vi "RPM_to_Motor_Input_v1.vi"(1 "Right Motor?":bool, 2 "RPM":dbl=1000.0) -> (0 "Motor Input":dbl)   [LabVIEW 2012]
uses:
  <vilib>/gmath/NI_Gmath.lvlib
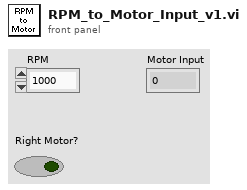
[diagram p1: front panel]
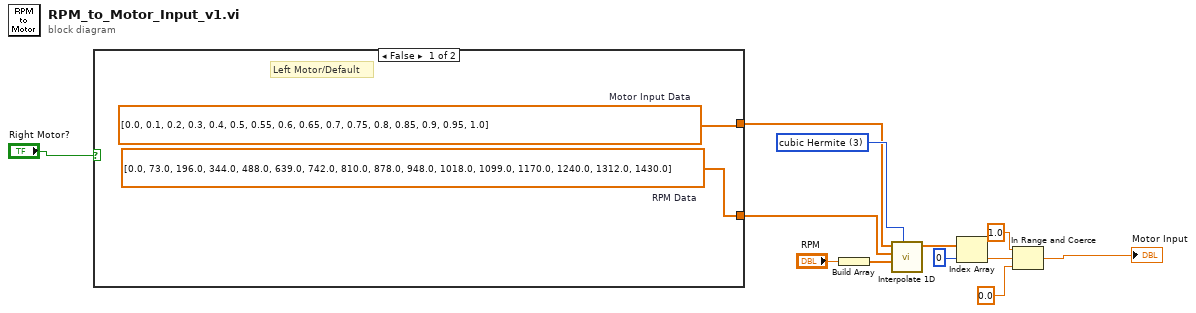
[diagram p0: block diagram]
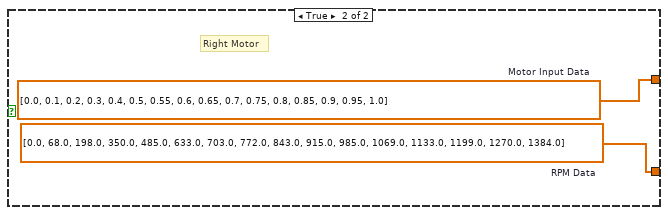
[diagram p2: hidden frame]
diagram:
  w8 = 3 items=["nearest", "linear", "spline", "cubic Hermite", "Lagrange"] ("method")
  n1 = case shown="False" "Right Motor?" {
    tunnel: [w14 w16] -> w6
    tunnel: [w13 w15] -> w5
    frame False {
      w14 = dbl[] [0.0, 0.1, 0.2, 0.3, 0.4, 0.5, 0.55, 0.6, 0.65, 0.7, 0.75, 0.8, 0.85, 0.9, 0.95, 1.0]  # Motor Input Data
      w13 = dbl[] [0.0, 73.0, 196.0, 344.0, 488.0, 639.0, 742.0, 810.0, 878.0, 948.0, 1018.0, 1099.0, 1170.0, 1240.0, 1312.0, 1430.0]  # RPM Data
      # "Left Motor/Default"
    }
    frame True {
      w16 = dbl[] [0.0, 0.1, 0.2, 0.3, 0.4, 0.5, 0.55, 0.6, 0.65, 0.7, 0.75, 0.8, 0.85, 0.9, 0.95, 1.0]  # Motor Input Data
      w15 = dbl[] [0.0, 68.0, 198.0, 350.0, 485.0, 633.0, 703.0, 772.0, 843.0, 915.0, 985.0, 1069.0, 1133.0, 1199.0, 1270.0, 1384.0]  # RPM Data
      # "Right Motor"
    }
  }
  n2 = Build Array("RPM") -> (w11:dbl[])
  n3 = call <vilib>:"Interpolate 1D.vi"("method"=w8, "xi"=w11, "X"=w5, "Y"=w6) -> ("yi"=w10:dbl[])  [unwired: 5 in, 2 out]
  n4 = Index Array(array=w10, index=0) -> (element=w7:dbl)
  n5 = In Range and Coerce(upper limit=1.0, x=w7, lower limit=0.0) -> (coerced(x)=→"Motor Input":dbl)  [unwired: 1 out]
